vi "OP UPH Config.vi"(8 "error in (no error)":errorcluster, 9 "UPH":T1[](array[typedef]), 10 "Enum":enum16{"init", "Read", "Write"}(ring)=enum."Read", 11 "Path":path) -> (0 "error out":errorcluster, 2 "UPH out":T1[](array[typedef]), 3 "Path out":path)   [LabVIEW 2014]
uses:
  <vilib>/Utility/xml.llb/Write to XML File(string).vi
  <vilib>/Utility/xml.llb/Read From XML File(string).vi
  Type'def/UPH Config.ctl
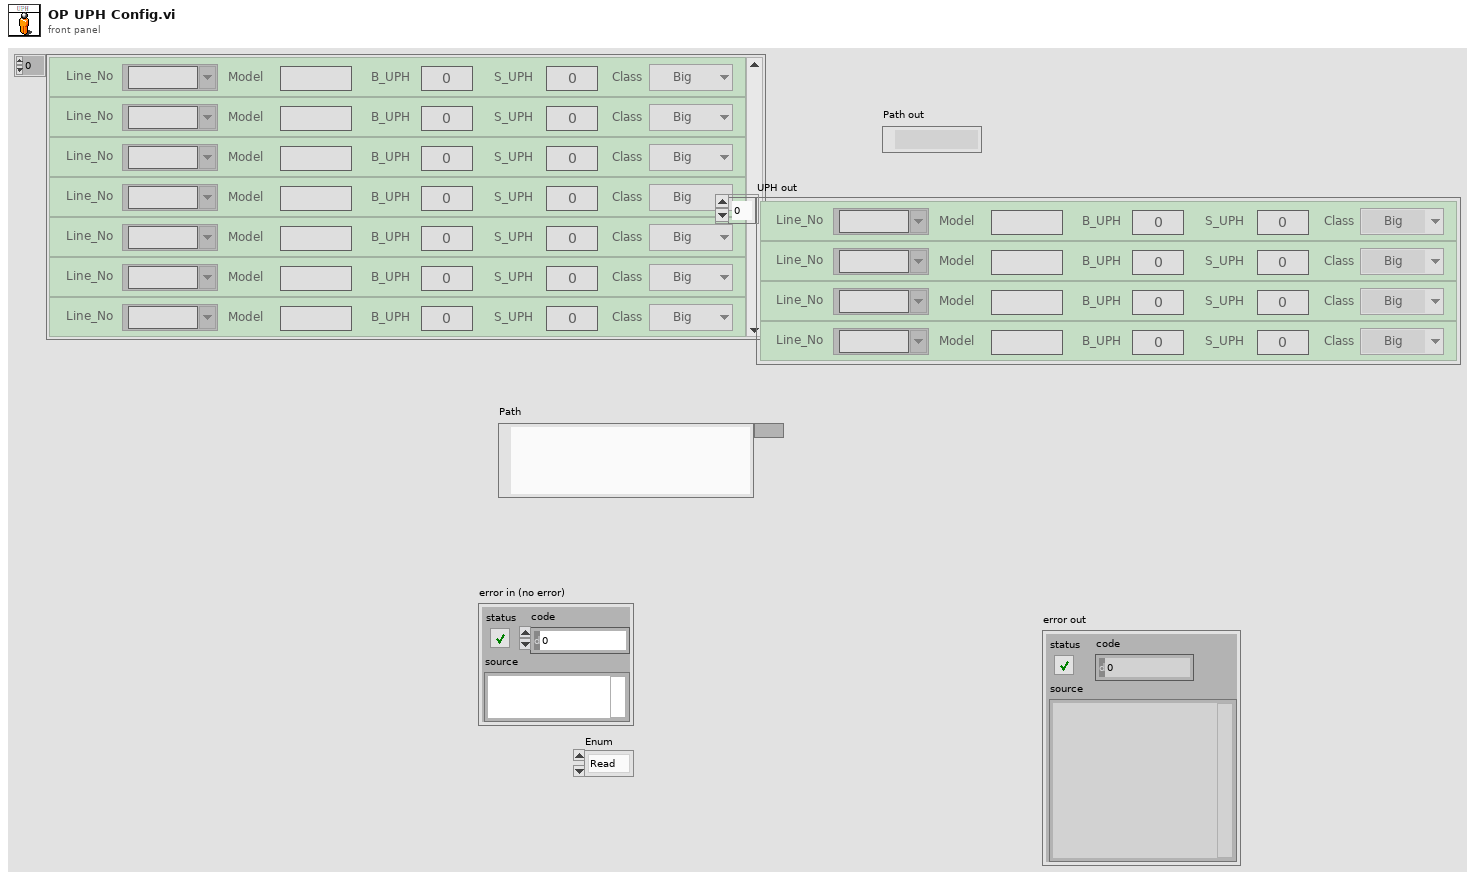
[diagram p1: front panel]
types:
  T1 = typedef "UPH Config.ctl" = cluster{"Line_No":string, "Model":string, "B_UPH ":i16, "S_UPH  ":i16, "Class":enum16{"Big", "Small"}}
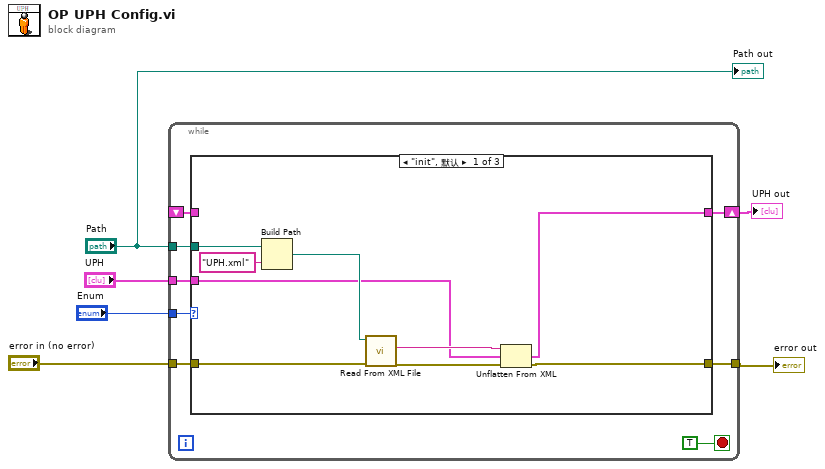
[diagram p0: block diagram]
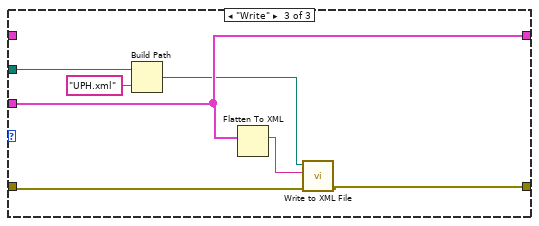
[diagram p3: hidden frame]
diagram:
  n1 = while {
    tunnel: "Enum" -> [w14]
    tunnel: "Path" -> [w13]
    tunnel: "error in (no error)" -> [w12]
    tunnel: "UPH" -> [w11]
    shift-right: [w10] -> w1
    shift-left: _ -> [w8]
    tunnel: [w9] -> w2
    stop <- TRUE stop-if-true
    n2 = case shown="\"init\", 默认" w14 {
      tunnel: w13 -> [w22 _ w31]
      tunnel: w12 -> [w21 w24 w26]
      tunnel: w11 -> [w18 _ w30]
      tunnel: [w15 w25 w30] -> w10
      tunnel: [w17 w24 w29] -> w9
      tunnel: w8 -> [_ w25 _]
      frame "init", Default {
        n3 = Build Path(base path=w22, name or relative path="UPH.xml") -> (appended path=w20:path)
        n4 = call-poly <vilib>:"Read From XML File.vi"("error in (no error)"=w21, "XML File Path"=w20) -> ("error out"=w16:errorcluster, "XML Elements"=w19:string)  [unwired: 7 in, 1 out]
        n5 = Unflatten From XML(xml string=w19, type=w18, error in (no error)=w16) -> (value=w15:T1[], error out=w17:errorcluster)
      }
      frame "Read" {
      }
      frame "Write" {
        n6 = Build Path(base path=w31, name or relative path="UPH.xml") -> (appended path=w28:path)
        n7 = Flatten To XML(anything=w30) -> (xml string=w27:string)
        n8 = call-poly <vilib>:"Write to XML File.vi"("error in (no error)"=w26, "XML Input"=w27, "XML File Path"=w28) -> ("error out"=w29:errorcluster)  [unwired: 6 in, 2 out]
      }
    }
  }
  "error out" <- w2
  "UPH out" <- w1
  "Path out" <- "Path"
